vi "Live.GetNodeAttribute.vi"(6 "timeout (5000 ms)":u32=5000, 8 "error in (no error)":errorcluster, 10 "node path":string, 11 "OPC UA client refnum in":refnum<k21>) -> (0 "error out":errorcluster, 1 "status":u32[](array[ring]) items=["Good"=0, "Bad_AttributeIdInvalid"=2153906176, "Bad_BrowseDirectionInvalid"=2152529920, "Bad_BrowseNameInvalid"=2153775104, "Bad_ContentFilterInvalid"=2152202240, "Bad_ContinuationPointInvalid"=2152333312, "Bad_DataEncodingInvalid"=2151153664, "Bad_DataEncodingUnsupported"=2151219200, "Bad_EventFilterInvalid"=2152136704, "Bad_FilterNotAllowed"=2152005632, "Bad_FilterOperandInvalid"=2160132096, "Bad_HistoryOperationInvalid"=2154889216, "Bad_HistoryOperationUnsupported"=2154954752, "Bad_IndexRangeInvalid"=2151022592, "Bad_IndexRangeNoData"=2151088128, "Bad_MonitoredItemFilterInvalid"=2151874560, "Bad_MonitoredItemFilterUnsupported"=2151940096, "Bad_MonitoredItemIdInvalid"=2151809024, "Bad_MonitoringModeInvalid"=2151743488, "Bad_NoCommunication"=2150694912, "Bad_NoContinuationPoints"=2152398848, "Bad_NodeClassInvalid"=2153709568, "Bad_NodeIdInvalid"=2150825984, "Bad_NodeIdUnknown"=2150891520, "Bad_NoDeleteRights"=2154364928, "Bad_NodeNotInView"=2152595456, "Bad_NotFound"=2151546880, "Bad_NotImplemented"=2151677952, "Bad_NotReadable"=2151284736, "Bad_NotSupported"=2151481344, "Bad_NotWritable"=2151350272, "Bad_ObjectDeleted"=2151612416, "Bad_OutOfRange"=2151415808, "Bad_ReferenceTypeIdInvalid"=2152464384, "Bad_SourceNodeIdInvalid"=2154037248, "Bad_StructureMissing"=2152071168, "Bad_TargetNodeIdInvalid"=2154102784, "Bad_TypeDefinitionInvalid"=2153971712, "Bad_TypeMismatch"=2155085824, "Bad_WaitingForInitialData"=2150760448], 2 "node attribute":T1={"name"="", "node type"=enum."Other", "DataType"=1, "access"=enum."Null", "description"=""} {"DataType" items=["Boolean"=1, "SByte"=2, "Byte"=3, "Int16"=4, "UInt16"=5, "Int32"=6, "UInt32"=7, "Int64"=8, "UInt64"=9, "Float"=10, "Double"=11, "String"=12, "DateTime"=13, "ByteString"=15, "Array of Boolean"=101, "Array of SByte"=102, "Array of Byte"=103, "Array of Int16"=104, "Array of UInt16"=105, "Array of Int32"=106, "Array of UInt32"=107, "Array of Int64"=108, "Array of UInt64"=109, "Array of Float"=110, "Array of Double"=111, "Array of String"=112, "Array of DateTime"=113, "Array of ByteString"=115]}, 3 "OPC UA client refnum out":refnum<k21>)   [LabVIEW 2013, in "OPC UA Client System Explorer.lvlib"]
uses:
  OPC UA Client System Explorer.lvlib
  <vilib>/OPCUA/client/ni_opcua_client.dll
  <resource>/objmgr/OpcUaClient.rc
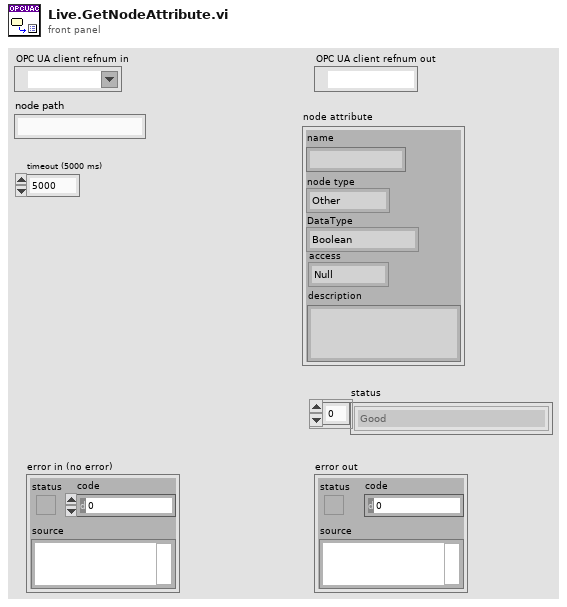
[diagram p1: front panel]
types:
  T1 = cluster{"name":string, "node type":enum32{"Other", "Folder", "Item/Property"}, "DataType":u32, "access":enum16{"Null", "Read", "Write", "Read&Write"}, "description":string}
  T2 = cluster{"displayName":string, "nodeType":i32, "dataType":u32, "accessLevel":u8, "description":string}
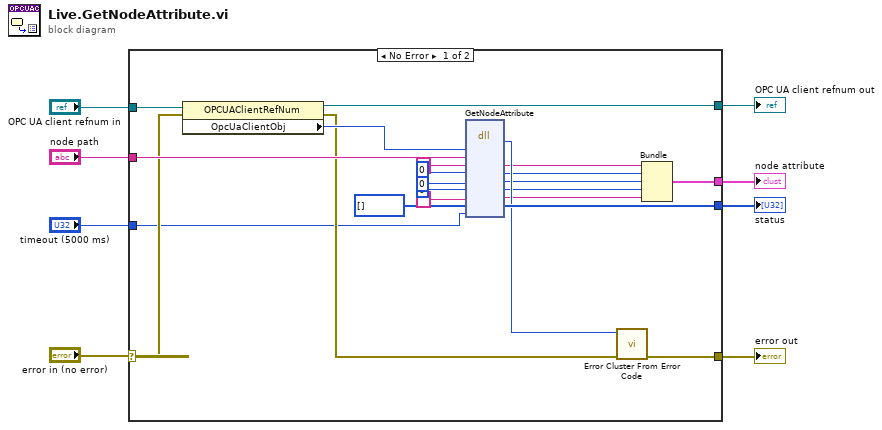
[diagram p0: block diagram]
diagram:
  n1 = case shown="No Error" "error in (no error)" {
    selector: "error in (no error)" -> [w16 w32]
    tunnel: "node path" -> [w30 _]
    tunnel: [w28 _] -> w7
    tunnel: [w27 w32] -> w5
    tunnel: [w20 _] -> w1
    tunnel: "OPC UA client refnum in" -> [w19 w31]
    tunnel: [w18 w31] -> w3
    tunnel: "timeout (5000 ms)" -> [w14 _]
    frame No Error {
      n2 = property class="OPCUAClientRefNum"(reference=w19, error in=w16) -> (reference out=w18:refnum<k21>, error out=w15:errorcluster, "OpcUaClientObj"=w17:i32)
      n3 = dll-call lib="C:/Program Files/National Instruments/LabVIEW 2013/vi.lib/OPCUA/client/ni_opcua_client.*" fn="GetNodeAttribute"("uaClientPtr"=w17, "nodeToRead"=w30, "displayName"="", "nodeType"=0, "dataType"=u32 0, "accessLevel"=u8 0, "description"="", "statusArray"=i32[] [] ("Array 2"), "timeout"=w14) -> ("return type"=w26:i32, "displayName"=w25:string, "nodeType"=w24:i32, "dataType"=w23:u32, "accessLevel"=w22:u8, "description"=w21:string, "statusArray"=w28:i32[])  [unwired: 6 in, 2 out]
      n4 = call <vilib>:"Error Cluster From Error Code.vi"("error in (no error)"=w15, "error code (0)"=w26) -> ("error out"=w27:errorcluster)  [unwired: 7 in]
      n5 = Bundle("displayName"=w25, "nodeType"=w24, "dataType"=w23, "accessLevel"=w22, "description"=w21) -> (w20:T2)  [unwired: 1 in]
    }
    frame Error {
    }
  }
  "error out" <- w5
  "node attribute" <- w1
  "status" <- w7
  "OPC UA client refnum out" <- w3
